vi "Core_[HSMS]Selected_Send Message.vi"(8 "error in (no error)":errorcluster, 10 "Command Data":T1, 11 "HSMS Class in":refnum<class "HSMS Class.lvclass">) -> (0 "error out":errorcluster, 3 "HSMS Class out":refnum<class "HSMS Class.lvclass">)   [LabVIEW 2020, in "SECS Communication.lvlib" / "HSMS Class.lvclass"]
uses:
  HSMS Class.lvclass
  Command Data.ctl
  SECS-II Class/SECS-II Class.lvclass
  Message Header.ctl
  PType.ctl
  SType.ctl
  Message Packet.ctl
  Notifier Type.ctl
  SECS-II Class/SECS-II Class.lvclass/SECS-II Class.ctl
  HSMS Class.lvclass/HSMS Class.ctl
  SECS-II Class/Read W-Bit.vi
  SECS-II Class/Read Function.vi
  SECS-II Class/Read System Btyes.vi
  Read Session ID.vi
  SECS-II Class/Write Message Header.vi
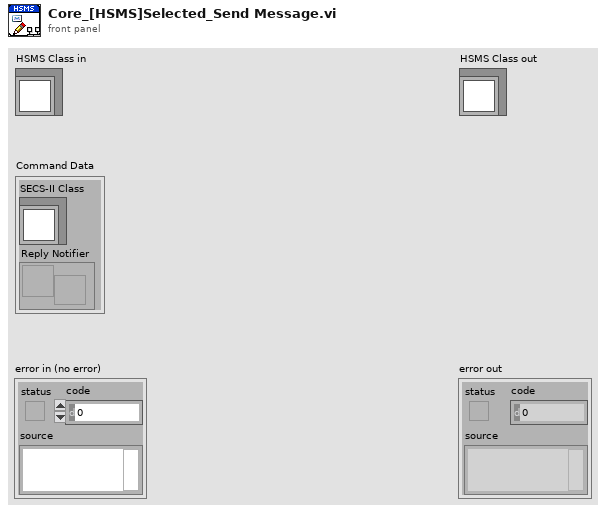
[diagram p1: front panel]
types:
  T1 = typedef "SECS Communication.lvlib/HSMS Class.lvclass/Command Data.ctl" = cluster{"SECS-II Class":refnum<class "SECS-II Class.lvclass">, "Reply Notifier":refnum<notifier>}
  T2 = typedef "SECS Communication.lvlib/HSMS Class.lvclass/Notifier Type.ctl" = enum16{"TCPIP Connect", "TCPIP Disconnect", "Receive Message", "Send Message", "T3 Timeout", "T6 Timeout", "T7 Timeout", "Error", "Stop"}
  T3 = typedef "SECS Communication.lvlib/HSMS Class.lvclass/Message Packet.ctl" = cluster{"Message Header Cluster":T4, "Message Header":u8[], "Message Text":u8[]}
  T4 = typedef "SECS Communication.lvlib/HSMS Class.lvclass/Message Header.ctl" = cluster{"Byte 0-1(Session ID)":u16, "W-Bit":bool, "Byte 2":u8, "Byte 3":u8, "Byte 4(PType)":T5, "Byte 5(SType)":T6, "Byte 6-9(System Btyes)":u8[]}
  T5 = typedef "SECS Communication.lvlib/HSMS Class.lvclass/PType.ctl" = enum8{"SECS-II Encoding", "Reserved"}
  T6 = typedef "SECS Communication.lvlib/HSMS Class.lvclass/SType.ctl" = enum8{"Data Message", "Select.req", "Select.rsp", "Deselect.req", "Deselect.rsp", "Linktest.req", "Linktest.rsp", "Reject.req", "Separate.req"}
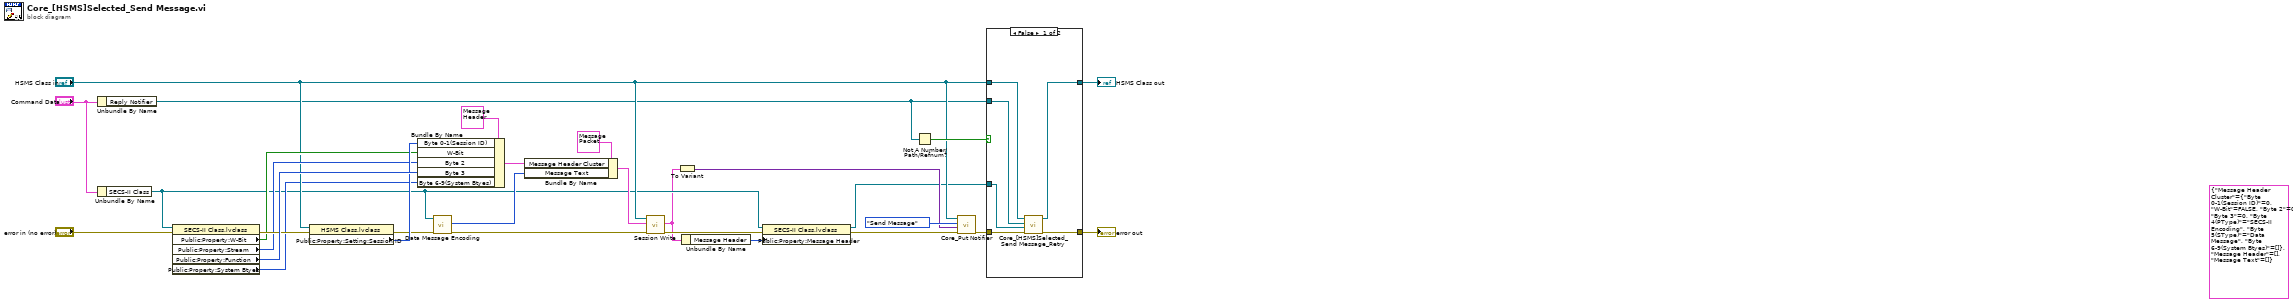
[diagram p0: block diagram]
diagram:
  (unwired) T3 {"Message Header Cluster"={"Byte 0-1(Session ID)"=0, "W-Bit"=FALSE, "Byte 2"=0, "Byte 3"=0, "Byte 4(PType)"=enum."SECS-II Encoding", "Byte 5(SType)"=enum."Data Message", "Byte 6-9(System Btyes)"=[]}, "Message Header"=[], "Message Text"=[]} ("Message Packet")
  n1 = Unbundle By Name("Command Data") -> ("Reply Notifier"=w8:refnum<notifier>)
  n2 = Unbundle By Name("Command Data") -> ("SECS-II Class"=w5:refnum<class "SECS-II Class.lvclass">)
  n3 = property class="SECS-II Class.lvclass"(reference=w5, error in="error in (no error)") -> (error out=w22:errorcluster, "Public:Property:W-Bit"=w18:bool, "Public:Property:Stream"=w19:u8, "Public:Property:Function"=w28:u8, "Public:Property:System Btyes"=w7:u8[])  [unwired: 1 out]
  n4 = property class="HSMS Class.lvclass"(reference="HSMS Class in", error in=w22) -> (error out=w21:errorcluster, "Public:Property:Setting:Session ID"=w23:u16)  [unwired: 1 out]
  n5 = Bundle By Name(cluster=T4 {"Byte 0-1(Session ID)"=0, "W-Bit"=FALSE, "Byte 2"=0, "Byte 3"=0, "Byte 4(PType)"=enum."SECS-II Encoding", "Byte 5(SType)"=enum."Data Message", "Byte 6-9(System Btyes)"=[]} ("Message Header"), "Byte 0-1(Session ID)"=w23, "W-Bit"=w18, "Byte 2"=w19, "Byte 3"=w28, "Byte 6-9(System Btyes)"=w7) -> (w26:T4)
  n6 = call "Data Message Encoding.vi"("error in"=w21, "SECS-II Class in"=w5) -> ("error out"=w24:errorcluster, "Message Text"=w25:u8[])  [unwired: 7 in, 1 out]
  n7 = Bundle By Name(cluster=T3 {"Message Header Cluster"={"Byte 0-1(Session ID)"=0, "W-Bit"=FALSE, "Byte 2"=0, "Byte 3"=0, "Byte 4(PType)"=enum."SECS-II Encoding", "Byte 5(SType)"=enum."Data Message", "Byte 6-9(System Btyes)"=[]}, "Message Header"=[], "Message Text"=[]} ("Message Packet"), "Message Header Cluster"=w26, "Message Text"=w25) -> (w11:T3)
  n8 = call "Session Write.vi"("error in (no error)"=w24, "Message Packet In"=w11, "HSMS Class in"="HSMS Class in") -> ("error out"=w6:errorcluster, "Message Packet Out"=w3:T3)  [unwired: 6 in, 1 out]
  n9 = To Variant(anything=w3) -> (Variant=w10:variant)
  n10 = Unbundle By Name(w3) -> ("Message Header"=w2:u8[])
  n11 = property class="SECS-II Class.lvclass"(reference=w5, error in=w6, "Public:Property:Message Header"=w2) -> (reference out=w1:refnum<class "SECS-II Class.lvclass">, error out=w4:errorcluster)
  n12 = Not A Number/Path/Refnum?(number/path/refnum=w8) -> (NaN/Path/Refnum?=w15:bool)
  n13 = call "Core_Put Notifier.vi"("error in (no error)"=w4, "Data"=w10, "Notifier Type"=Notifier_Type."Send Message", "HSMS Class in"="HSMS Class in") -> ("error out"=w9:errorcluster)  [unwired: 6 in, 1 out]
  n14 = case shown="False" w15 {
    tunnel: w9 -> [w35 w37]
    tunnel: "HSMS Class in" -> [w32 w36]
    tunnel: [w30 w37] -> w16
    tunnel: w8 -> [w33 _]
    tunnel: [w31 w36] -> w14
    tunnel: w1 -> [w34 _]
    frame False {
      n15 = call "Core_[HSMS]Selected_Send Message_Retry.vi"("error in (no error)"=w35, "SECS-II Class"=w34, "Reply Notifier"=w33, "HSMS Class in"=w32) -> ("error out"=w30:errorcluster, "HSMS Class out"=w31:refnum<class "HSMS Class.lvclass">)  [unwired: 6 in]
    }
    frame True {
    }
  }
  "error out" <- w16
  "HSMS Class out" <- w14
